vi "ExEMCircBufROI.vi"() -> ()   [LabVIEW 2010]
uses:
  CamHandle.vi
panel:
  in  "av gain":dbl format="%.2f"
  in  "Invert Logic output":bool
  in  "Logic Output":i32
  in  "Fan":i32=1
  in  "ADC Gain":u32
  out "ADC Speed (Khz)":u32
  in  "Fast ADC":bool
  in  "X Start":u32=1 min=1 step=1
  in  "Y Bin":u32=1 min=1 step=1
  in  "X End":u32=512 min=1 max=512 step=1
  in  "X Bin":u32=1 min=1 step=1
  in  "Y Start":u32=1 min=1 step=1
  in  "Y End":u32=512 min=1 max=512 step=1
  in  "Temperature":dbl=-55.0 format="%.2f"
  in  "Exposure":dbl min=0.0 step=0.001 format="%.3f"
  in  "stop":bool
  in  "Store":bool
  out "error out":errorcluster
  in  "error in (no error)":errorcluster
  # "ExEMCircBufROI:\nThis example allows a single ROI\nto be programmed up. It then runs\nin sync (focus) mode displaying \nthe ROI data as it comes in.\nNote: this example requires the \ncamera support circular buffers.\nThis example also shows how to \nsetup the cascade to run in over-\nlapped mode and how to set the\non-chip multiplication gain and how\nto set the readout port."
  # "Warning: you must open and run once the VI ExOpenGlobalCam.vi.\nYou only need to run it once then you can run this Example VI as many\ntimes as you want."
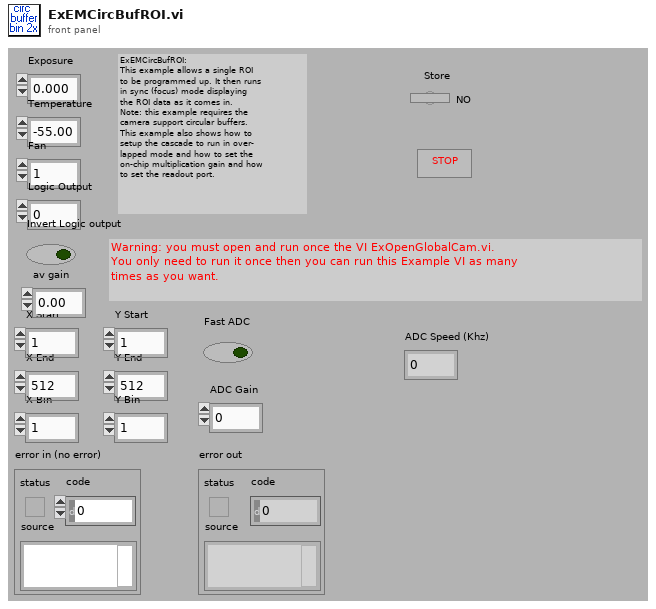
[diagram p1: front panel]
types:
  T1 = cluster{"X Start":u32, "X End":u32, "X Bin":u32, "Y Start":u32, "Y End":u32, "Y Bin":u32}
  T2 = cluster{"acquire focus mode":u32, "Exposure":dbl, "Number of Images":u32, "Software accumulation":u32}
  T3 = cluster{"Camera Handle":u32, "File Handle":u32, "Display Handle":u32, "Image Handle":u32}
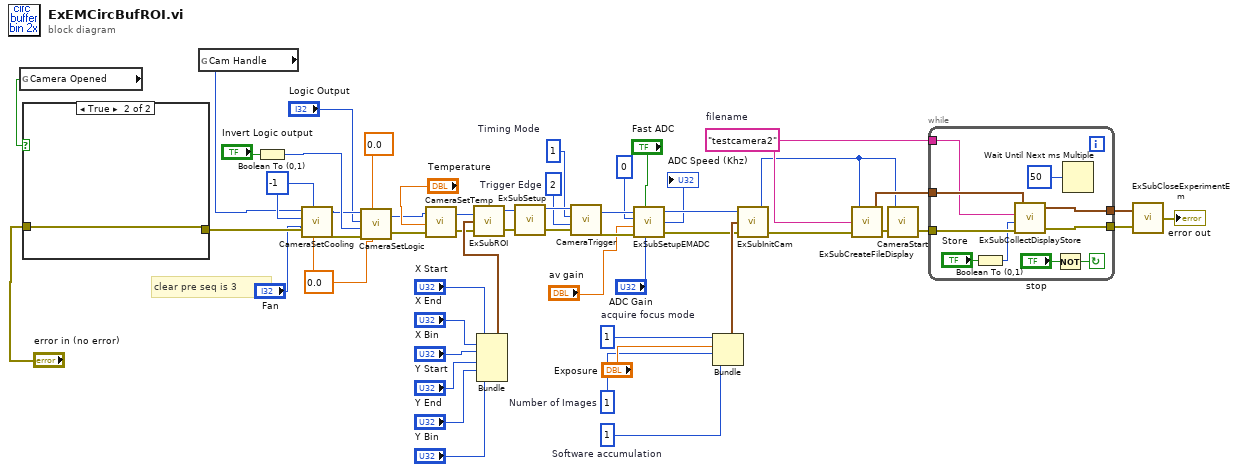
[diagram p0: block diagram]
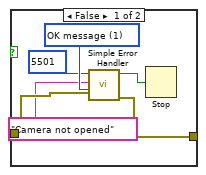
[diagram p2: hidden frame]
diagram:
  w5 = 0.0
  w6 = -1
  w39 = u32 1  # Timing Mode
  w40 = u32 2  # Trigger Edge
  w43 = u32 1  # acquire focus mode
  w42 = u32 1  # Number of Images
  w41 = u32 1  # Software accumulation
  w54 = "testcamera2"  # filename
  # "clear pre seq is 3"
  n1 = global read "CamHandle.vi" "Camera Opened"() -> (w15:bool)
  n2 = case shown="True" w15 {
    tunnel: "error in (no error)" -> [w59 w61]
    tunnel: [w58 w61] -> w13
    frame False {
      w60 = u16 1 items=["no dialog", "OK message", "continue or stop message"] ("type of dialog (OK msg:1)")
      n3 = call <vilib>:"Simple Error Handler.vi"("error code (no error:0)"=5501, "error source (\" \")"="Camera not opened", "type of dialog (OK msg:1)"=w60, "error in (no error)"=w59) -> ("error?"=w56:bool, "error out"=w58:errorcluster)  [unwired: 1 in, 3 out]
      n4 = Stop(stop? (T)=w56) -> ()
    }
    frame True {
    }
  }
  n5 = global read "CamHandle.vi" "Cam Handle"() -> (w1:u32)
  n6 = Boolean To (0,1)(Boolean="Invert Logic output") -> (0, 1=w9:i16)
  n7 = call <userlib>:"CameraSetCooling.vi"("Reserved"=w5, "Cooling Mode"=w6, "error in (no error)"=w13, "Fan"="Fan", "Cooling"=w6, "Camera Handle"=w1) -> ("error out"=w12:errorcluster, "Camera Handle"=w8:u32)
  n8 = call <userlib>:"CameraSetLogic.vi"("Reserved 2"=w5, "Reserved"=0.0, "error in (no error)"=w12, "Invert Logic"=w9, "Logic Output"="Logic Output", "Camera Handle"=w8) -> ("error out"=w11:errorcluster, "Camera Handle"=w4:u32)
  n9 = call <userlib>:"CameraSetTemp.vi"("error in (no error)"=w11, "Temperature"="Temperature", "Camera Handle"=w4) -> ("error out"=w29:errorcluster, "Camera Handle"=w28:u32)
  n10 = Bundle("X Start"="X Start", "X End"="X End", "X Bin"="X Bin", "Y Start"="Y Start", "Y End"="Y End", "Y Bin"="Y Bin") -> (w31:T1)  [unwired: 1 in]
  n11 = call "ExSubROI.vi"("error in (no error)"=w29, "ROI"=w31, "Camera Handle"=w28) -> ("error out"=w26:errorcluster, "Camera Handle"=w30:u32)
  n12 = call "ExSubSetup.vi"("error in (no error)"=w26, "Camera Handle"=w30) -> ("error out"=w25:errorcluster, "Camera Handle"=w46:u32)
  n13 = call <userlib>:"CameraTrigger.vi"("error in"=w25, "Trigger Edge"=w40, "Timing Mode"=w39, "Camera Handle"=w46) -> ("error out"=w23:errorcluster, "Camera Handle"=w24:u32)
  n14 = call "ExSubSetupEMADC.vi"("Camera Handle"=w24, "Fast ADC"="Fast ADC", "ReadOut Port"=0, "Avalanche Gain\nOnly valid for \nport 0"="av gain", "ADC Gain"="ADC Gain", "error in (no error)"=w23) -> ("Camera Handle"=w21:u32, "ADC Speed (Khz)"=→"ADC Speed (Khz)":u32, "error out"=w22:errorcluster)
  n15 = Bundle("acquire focus mode"=w43, "Exposure"="Exposure", "Number of Images"=w42, "Software accumulation"=w41) -> (w52:T2)  [unwired: 1 in]
  n16 = call "ExSubInitCam.vi"("error in (no error)"=w22, "Camera Information"=w52, "Camera Handle"=w21) -> ("error out"=w51:errorcluster, "Camera Handle"=w38:u32)
  n17 = call "ExSubCreateFileDisplay.vi"("error in (no error)"=w51, "File and Display Name"=w54, "Camera Handle"=w38) -> ("error out"=w44:errorcluster, "Handles Out"=w50:T3)
  n18 = call <userlib>:"CameraStart.vi"("error in"=w44, "Camera Handle"=w38) -> ("error out"=w45:errorcluster)  [unwired: 1 out]
  n19 = while {
    tunnel: w50 -> [w70]
    tunnel: w45 -> [w69]
    tunnel: w54 -> [w62]
    tunnel: [w67] -> w48
    tunnel: [w68] -> w49
    stop <- w65 continue-if-true
    n20 = Boolean To (0,1)(Boolean="Store") -> (0, 1=w63:i16)
    n21 = call "ExSubCollectDisplayStore.vi"("error in (no error)"=w69, "Store flag"=w63, "Display Title"=w62, "Handle Cluster"=w70) -> ("error out"=w67:errorcluster, "Handle Cluster Out"=w68:T3)  [unwired: 1 out]
    n22 = Not(x="stop") -> (.not. x?=w65:bool)
    n23 = Wait Until Next ms Multiple(millisecond multiple=u32 50) -> ()  [unwired: 1 out]
  }
  n24 = call "ExSubCloseExperimentEm.vi"("error in (no error)"=w48, "Handles In"=w49) -> ("error out"=→"error out":errorcluster)
